vi "Flatten Value.vi"(8 "Error In":errorcluster, 11 "Bool In":refnum<class "Bool.lvclass">) -> (0 "Error Out":errorcluster, 1 "Value":string, 3 "Bool Out":refnum<class "Bool.lvclass">)   [LabVIEW 2017, in "Tree API.lvlib" / "Bool.lvclass"]
uses:
  Bool.lvclass
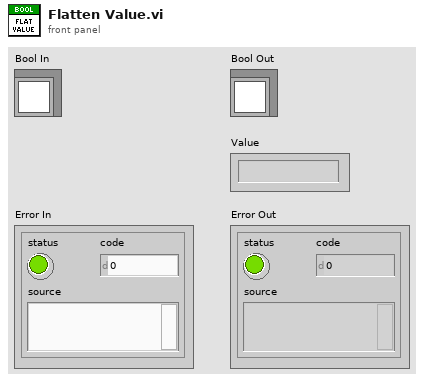
[diagram p1: front panel]
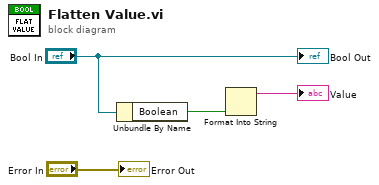
[diagram p0: block diagram]
diagram:
  n1 = Unbundle By Name("Bool In") -> ("Boolean"=w3:bool)
  n2 = Format Into String(w3) -> (resulting string=→"Value":string)  [unwired: 3 in, 1 out]
  "Bool Out" <- "Bool In"
  "Error Out" <- "Error In"
